vi "String (RAW) To String.vi"(7 "Raw String to String? [T]":bool=TRUE, 8 "error in (no error)":errorcluster, 10 "String (RAW)":string, 11 "Registry Object":refnum<class "Carya Config.lvclass">) -> (0 "error out":errorcluster, 2 "String":string, 3 "Registry Object":refnum<class "Carya Config.lvclass">)   [LabVIEW 2013, in "Carya Config.lvclass"]
doc: "Copyright 2018, Carya Automatisering, Wiebe Walstra."
uses:
  Carya Config.lvclass
  <vilib>/regexp/Match Regular Expression.xnode
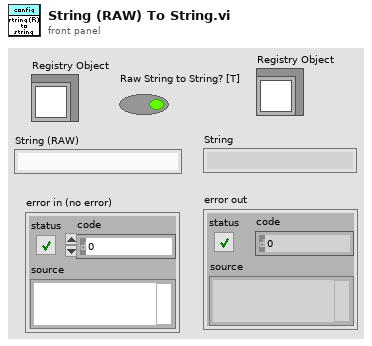
[diagram p1: front panel]
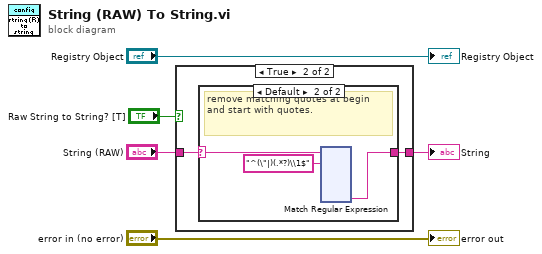
[diagram p0: block diagram]
diagram:
  n1 = case shown="True" "Raw String to String? [T]" {
    tunnel: [w6 w8] -> w3
    tunnel: "String (RAW)" -> [w6 w7]
    frame False {
    }
    frame True {
      n2 = case shown="Default" w7 {
        selector: w7 -> [w9 w12]
        tunnel: [w9 w10] -> w8
        frame "", "\"" {
          # "\" stays \""
        }
        frame Default {
          # "remove matching quotes at begin and start with quotes."
          n3 = xnode "Match Regular Expression"("input string"=w12, "regular expression"="^(\"|)(.*?)\\1$") -> ("submatch 2"=w10:string)  [unwired: 4 in, 6 out]
        }
      }
    }
  }
  "String" <- w3
  "Registry Object" <- "Registry Object"
  "error out" <- "error in (no error)"
